vi "Read FPPos.vi"(3 "FP":refnum<class "DecFrame_FP.lvclass">) -> (1 "FPPos Out":refnum<class "FPPos.lvclass">)   [LabVIEW 2024, in "DecFrame_FP.lvclass"]
uses:
  DecFrame_FP/DecFrame_FP.lvclass
  FPPos/FPPos.lvclass
  DecFrame_FP/DecFrame_FP.lvclass/DecFrame_FP.ctl
  Frame_FPPos/Frame_FPPos.lvclass
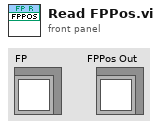
[diagram p1: front panel]
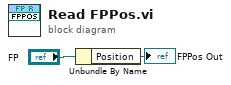
[diagram p0: block diagram]
diagram:
  n1 = Unbundle By Name("FP") -> ("Position"=→"FPPos Out":refnum<class "Frame_FPPos.lvclass">)
